vi "PathPlanner_PathFinder_DoMinor.vi"   [LabVIEW 2019]
uses:
  PathPlannerLib24/VI/PathPlanner_PathFinder_TopKey.vi
  PathPlannerLib24/VI/PathPlanner_PathFinder_ComparePair.vi
  PathPlannerLib24/VI/PathPlanner_PathFinder_Key.vi
  PathPlannerLib24/VI/PathPlanner_GridPosition_HashCode.vi
  PathPlannerLib24/VI/PathPlanner_PathFinder_UpdateState.vi
  PathPlannerLib24/VI/PathPlanner_PathFinder_GetOpenNeighbors.vi
  PathPlannerLib24/VI/PathPlanner_GridPosition_Equals.vi
  PathPlannerLib24/VI/PathPlanner_PathFinder_GridPosToTranslation2d.vi
  <vilib>/Rock Robotics/WPI/ThirdParty/JAS_Junk/TrajLib/Translation2d_GetDistance.vi
  PathPlannerLib24/VI/PathPlanner_PathFinder_Constants.vi
  <vilib>/Rock Robotics/WPI/ThirdParty/JAS_Junk/TrajLib/Translation2d_Create_DistAng.vi
  <vilib>/Rock Robotics/WPI/ThirdParty/JAS_Junk/TrajLib/Translation2d_Minus.vi
  <vilib>/Rock Robotics/WPI/ThirdParty/JAS_Junk/TrajLib/Translation2d_GetAngle.vi
  <vilib>/Rock Robotics/WPI/ThirdParty/JAS_Junk/TrajLib/Translation2d_Plus.vi
  PathPlannerLib24/VI/PathPlanner_PathFinder_ExtractPathSub1ALT.vi
  PathPlannerLib24/VI/PathPlanner_PathFinder_IsWalkable.vi
  PathPlannerLib24/VI/PathPlanner_GridPosition_FromHash.vi
  PathPlannerLib24/VI/PathPlanner_PathFinder_Heuristic.vi
  PathPlannerLib24/VI/PathPlanner_GridPosition_Get.vi
  PathPlannerLib24/VI/PathPlanner_PathFinder_Cost.vi
  PathPlannerLib24/VI/PathPlanner_GridPosition_New.vi
  <vilib>/Rock Robotics/WPI/ThirdParty/JAS_Junk/TrajLib/Translation2d_Create.vi
  <vilib>/Rock Robotics/WPI/ThirdParty/JAS_Junk/TrajLib/Util_CalcDist.vi
  <vilib>/Rock Robotics/WPI/ThirdParty/JAS_Junk/TrajLib/Rotation2d_GetAngleCosSin.vi
  <vilib>/Rock Robotics/WPI/ThirdParty/JAS_Junk/TrajLib/Translation2d_GetXY.vi
  <vilib>/Rock Robotics/WPI/ThirdParty/JAS_Junk/TrajLib/Rotation2d_CreateXY.vi
  PathPlannerLib24/VI/PathPlanner_PathFinder_IsCollision.vi
  PathPlannerLib24/VI/PathPlanner_GridPosition_Print.vi
  <vilib>/robotics/Navigation/shared/MapNode/AbstractDstarNode/NI_Robotics_AbstractDstarNode.lvclass
  C:/Program Files/National Instruments/LabVIEW 2019/vi.lib/robotics/Navigation/shared/MapNode/AbstractAstarNode/NI_Robotics_AbstractAstarNode.lvclass
  PathPlannerLib24/VI/PathPlanner_PathFinder_Globals.vi
  <vilib>/robotics/Navigation/shared/WorldMap/OccupancyGridWorldMap/Get Cells in Path.vi
  PathPlannerLib24/VI/PathPlanner_PathFinder_ApplyControlSmooth.vi
  PathPlannerLib24/VI/PathPlanner_PathFinder_ApplyAnchorSmooth.vi
  PathPlannerLib24/PathPlanner24.lvlib
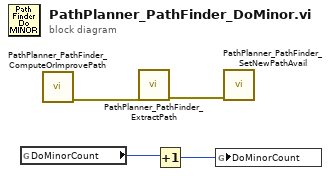
[diagram p0: block diagram]
diagram:
  n1 = global read "PathPlanner_PathFinder_Globals.vi" "DoMinorCount"() -> (w2:i64)
  n2 = call "PathPlanner_PathFinder_ComputeOrImprovePath.vi"() -> ("error out"=w4:errorcluster)  [unwired: 11 in]
  n3 = call "PathPlanner_PathFinder_ExtractPath.vi"("error in (no error)"=w4) -> ("error out"=w3:errorcluster)  [unwired: 10 in]
  n4 = Increment(x=w2) -> (x+1=w1:i64)
  n5 = global write "PathPlanner_PathFinder_Globals.vi" "DoMinorCount"(w1) -> ()
  n6 = call "PathPlanner_PathFinder_SetNewPathAvail.vi"("error in (no error)"=w3) -> ()  [unwired: 10 in, 1 out]
